vi "run.vi"(8 "results reporter":refnum<class "results reporter.lvclass">, 9 "execution system":T1=enum."standard", 10 "thread pool":refnum<class "thread pool.lvclass">, 11 "task in":refnum<class "task.lvclass">) -> (2 "result":refnum<class "result.lvclass">, 3 "task out":refnum<class "task.lvclass">)   [LabVIEW 2014, in "task.lvclass"]
uses:
  task.lvclass
  result/result.lvclass
  dispatcher/thread pool.lvclass
  dispatcher/execution system.ctl
  results reporter/results reporter.lvclass
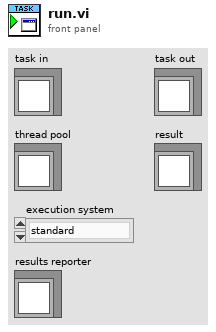
[diagram p1: front panel]
types:
  T1 = typedef "thread pool.lvclass/execution system.ctl" = enum32{"user interface", "standard", "instrument i/o", "data acquisition", "other 1", "other 2"}
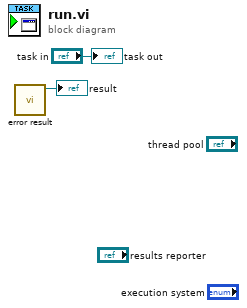
[diagram p0: block diagram]
diagram:
  n1 = call "error result.vi"() -> ("result"=→"result":refnum<class "result.lvclass">)  [unwired: 11 in]
  "task out" <- "task in"
